vi "GetData.vi"(0 "reference":refnum<class "VdRs232.lvclass">, 1 "stringIn":string, 2 "numberOfBytes(-1=all)":i32=-1, 3 "timeOut(-1ms=ignored)":i32=-1, 4 "MatchPatternToIndicateCompleteResponse(Use default if not wired)":string, 5 "error in (no error)":errorcluster, 6 "WaitForOtherProcessesToBeFinished(False)":bool, 9 "WaitTimeIfPatternNotFound(20ms)":u32=20) -> (14 "duplicate reference":refnum<class "VdRs232.lvclass">, 15 "wholeString":string, 16 "stringRead":string, 17 "TimedOut":bool, 19 "error out":errorcluster)   [LabVIEW 2020, in "VdRs232.lvclass"]
doc: "Reads data from the com-port"
uses:
  VdRs232.lvclass
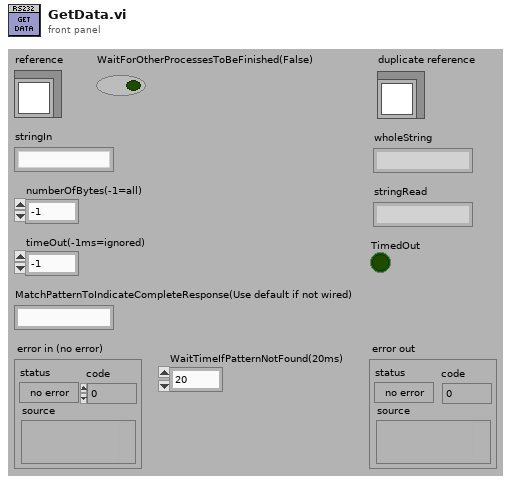
[diagram p1: front panel]
types:
  T1 = typedef "VdRs232.lvclass/ObjectAttributes.ctl" = cluster{"visaRef":refnum<visa-resource-name>, "portSetting":T2, "TimeoutTime(ms)":u32, "TerminationCharUsed":bool, "MatchPatternToIndicateCompleteResponse":string, "Creators":i32, "EndCharToSendForEveryMessage":string, "DefaultReadDataSize":u32, "SynchronousMode":bool, "Lock":T7}
  T2 = typedef "VdRs232.lvclass/ComParamsType.ctl" = cluster{"portNbr":T3, "baudRate":T4, "flowControl":T5, "parity":T6, "dataBits":u16, "stop bits (10: 1 bit)":u16}
  T3 = typedef "VdRs232.lvclass/VdRs232I_ComPortType.ctl" = enum16{"Com1", "Com2", "Com3", "Com4", "Com5", "Com6", "Com7", "Com8", "Com9", "Com10", "Com11", "Com12", "Com13", "Com14", "Com15", "Com16", "Com17", "Com18", "Com19", "Com20", "Com21", "Com22", "Com23", "Com24", "Com25", "Com26", "Com27", "Com28", "Com29", "Com30", "Com31", "Com32", "Com33", "Com34", "Com35", "Com36", "Com37", "Com38", "Com39", "Com40", "Com41", "Com42", "Com43", "Com44", "Com45", "Com46", "Com47", "Com48", "Com49", "Com50", "Com51", "Com52", "Com53", "Com54", "Com55", "Com56", "Com57", "Com58", "Com59", "Com60", "Com61", "Com62", "Com63", "Com64", "Com65", "Com66", "Com67", "Com68", "Com69", "Com70", "Com71", "Com72", "Com73", "Com74", "Com75", "Com76", "Com77", "Com78", "Com79", "Com80", "Com81", "Com82", "Com83", "Com84", "Com85", "Com86", "Com87", "Com88", "Com89", "Com90", "Com91", "Com92", "Com93", "Com94", "Com95", "Com96", "Com97", "Com98", "Com99", "Com100", "Com101", "Com102", "Com103", "Com104", "Com105", "Com106", "Com107", "Com108", "Com109", "Com110", "Com111", "Com112", "Com113", "Com114", "Com115", "Com116", "Com117", "Com118", "Com119", "Com120", "Com121", "Com122", "Com123", "Com124", "Com125", "Com126", "Com127", "Com128", "Com129", "Com130", "Com131", "Com132", "Com133", "Com134", "Com135", "Com136", "Com137", "Com138", "Com139", "Com140", "Com141", "Com142", "Com143", "Com144", "Com145", "Com146", "Com147", "Com148", "Com149", "Com150", "Com151", "Com152", "Com153", "Com154", "Com155", "Com156", "Com157", "Com158", "Com159", "Com160", "Com161", "Com162", "Com163", "Com164", "Com165", "Com166", "Com167", "Com168", "Com169", "Com170", "Com171", "Com172", "Com173", "Com174", "Com175", "Com176", "Com177", "Com178", "Com179", "Com180", "Com181", "Com182", "Com183", "Com184", "Com185", "Com186", "Com187", "Com188", "Com189", "Com190", "Com191", "Com192", "Com193", "Com194", "Com195", "Com196", "Com197", "Com198", "Com199", "Com200", "Com201", "Com202", "Com203", "Com204", "Com205", "Com206", "Com207", "Com208", "Com209", "Com210", "Com211", "Com212", "Com213", "Com214", "Com215", "Com216", "Com217", "Com218", "Com219", "Com220", "Com221", "Com222", "Com223", "Com224", "Com225", "Com226", "Com227", "Com228", "Com229", "Com230", "Com231", "Com232", "Com233", "Com234", "Com235", "Com236", "Com237", "Com238", "Com239", "Com240", "Com241", "Com242", "Com243", "Com244", "Com245", "Com246", "Com247", "Com248", "Com249", "Com250", "Com251", "Com252", "Com253", "Com254", "Com255"}
  T4 = typedef "VdRs232.lvclass/VdBaudRateType.ctl" = enum16{"1200", "2400", "9600", "14400", "19200", "28800", "38400", "57600", "115200", "230400", "460800", "691200", "921600"}
  T5 = typedef "VdRs232.lvclass/VdFlowControlType.ctl" = enum16{"None", "CTS/RTS", "XOn/XOff"}
  T6 = typedef "VdRs232.lvclass/VdParityType.ctl" = enum16{"None", "Odd", "Even"}
  T7 = typedef "Semaphore RefNum" = refnum<k1>
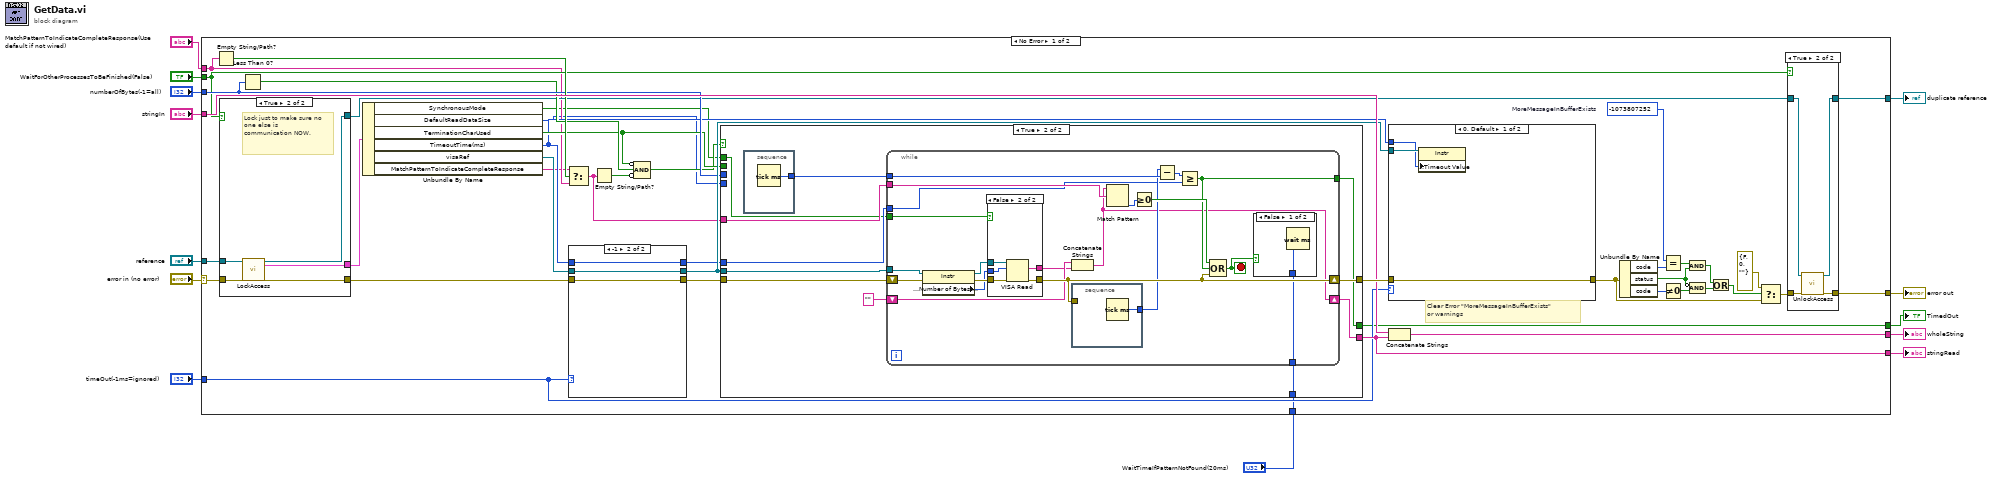
[diagram p0: block diagram]
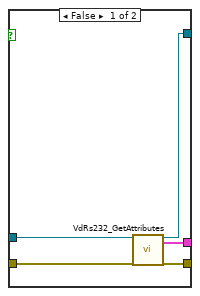
[diagram p3: hidden frame]
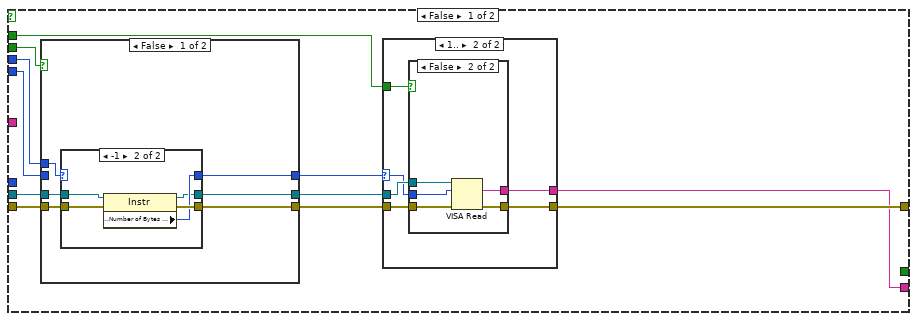
[diagram p4: hidden frame]
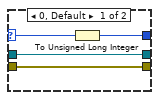
[diagram p5: hidden frame]
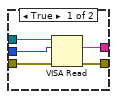
[diagram p8: hidden frame]
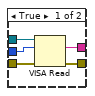
[diagram p9: hidden frame]
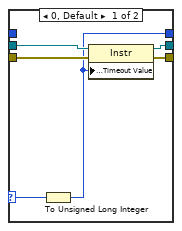
[diagram p12: hidden frame]
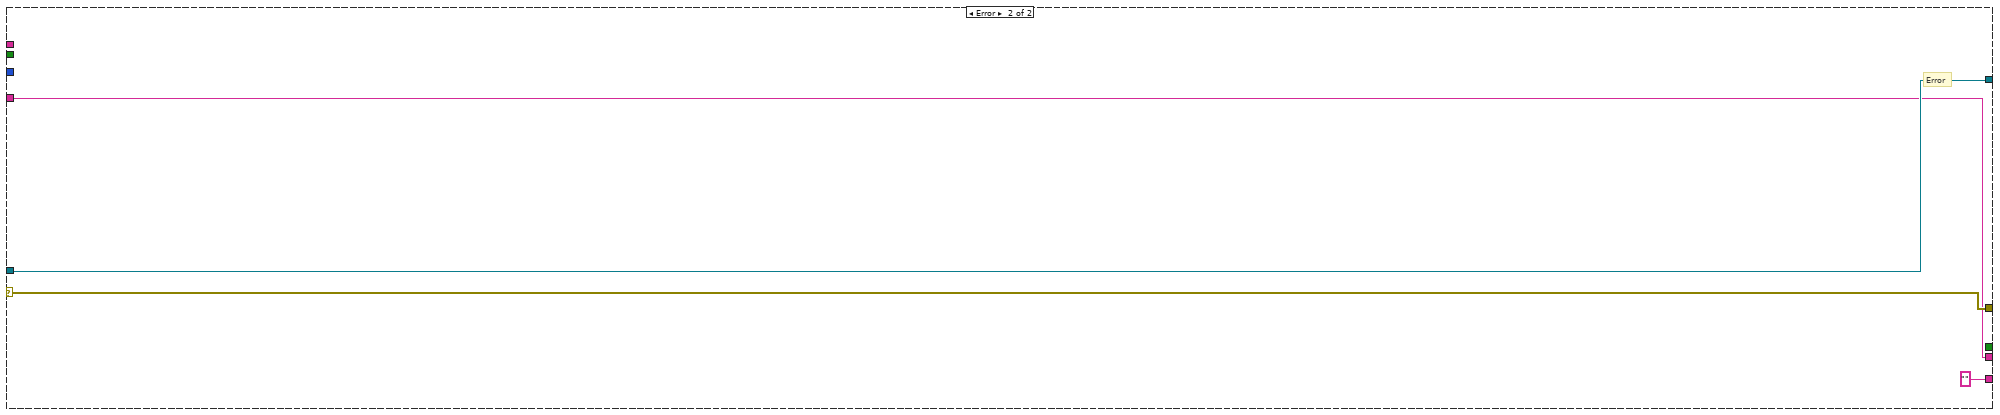
[diagram p13: hidden frame]
diagram:
  n1 = case shown="No Error" "error in (no error)" {
    selector: "error in (no error)" -> [w52 w179]
    tunnel: [w49 w179] -> w13
    tunnel: "reference" -> [w23 w178]
    tunnel: [w21 w178] -> w10
    tunnel: "numberOfBytes(-1=all)" -> [w32 _]
    tunnel: [w46 "" ("read buffer")] -> w7
    tunnel: "timeOut(-1ms=ignored)" -> [w43 _]
    tunnel: "stringIn" -> [w47 w176]
    tunnel: [w45 w176] -> w5
    tunnel: "MatchPatternToIndicateCompleteResponse(Use default if not wired)" -> [w18 _]
    tunnel: [w24 _] -> w3
    tunnel: "WaitForOtherProcessesToBeFinished(False)" -> [w19 _]
    tunnel: "WaitTimeIfPatternNotFound(20ms)" -> [w14 _]
    frame No Error {
      w41 = -1073807252  # MoreMessageInBufferExists
      # "Clear Error \"MoreMessageInBufferExists\"\nor warnings"
      n2 = Empty String/Path?(string/path=w18) -> (empty?=w33:bool)
      n3 = case shown="True" w19 {
        tunnel: w23 -> [w65 w70]
        tunnel: w52 -> [w67 w72]
        tunnel: [w66 w71] -> w51
        tunnel: [w64 w69] -> w22
        tunnel: [w63 w68] -> w20
        frame False {
          n4 = call "VdRs232_GetAttributes.vi"("reference in"=w65, "error in (no error)"=w67) -> ("reference out"=w64:refnum<class "VdRs232.lvclass">, "Data"=w63:T1, "error out"=w66:errorcluster)  [unwired: 1 in, 14 out]
        }
        frame True {
          # "Lock just to make sure no one else is communication NOW."
          n5 = call "LockAccess.vi"("reference in"=w70, "error in (no error)"=w72) -> ("reference out"=w69:refnum<class "VdRs232.lvclass">, "Data"=w68:T1, "error out"=w71:errorcluster)  [unwired: 14 in, 1 out]
        }
      }
      n6 = Less Than 0?(x=w32) -> (x < 0?=w31:bool)
      n7 = Unbundle By Name(w20) -> ("SynchronousMode"=w15:bool, "DefaultReadDataSize"=w16:u32, "TerminationCharUsed"=w30:bool, "TimeoutTime(ms)"=w26:u32, "visaRef"=w48:refnum<visa-resource-name>, "MatchPatternToIndicateCompleteResponse"=w17:string)
      n8 = Select(t=w17, s=w33, f=w18) -> (s? t:f=w28:string)
      n9 = case shown="-1" w43 {
        selector: w43 -> [w168 _]
        tunnel: [w172 w175] -> w56
        tunnel: w51 -> [w171 w175]
        tunnel: [w170 w174] -> w44
        tunnel: w48 -> [w169 w174]
        tunnel: w26 -> [_ w173]
        tunnel: [w167 w173] -> w25
        frame 0, Default {
          n10 = To Unsigned Long Integer(number=w168) -> (unsigned 32bit integer=w167:u32)
          n11 = property class="Instr"(reference=w169, error in=w171, "General Settings:Timeout Value"=w167) -> (reference out=w170:refnum<visa-resource-name>, error out=w172:errorcluster)
        }
        frame -1 {
        }
      }
      n12 = Empty String/Path?(string/path=w28) -> (empty?=w27:bool)
      n13 = Compound Arithmetic op=AND(invert w30, w31, invert w27) -> (w29:bool)
      n14 = case shown="True" w29 {
        tunnel: w56 -> [w83 w128]
        tunnel: [w80 w125] -> w46
        tunnel: [w81 w129] -> w55
        tunnel: w44 -> [w77 w124]
        tunnel: w32 -> [w76 _]
        tunnel: w30 -> [w75 _]
        tunnel: w28 -> [_ w123]
        tunnel: w25 -> [_ w122]
        tunnel: [_ w121] -> w24
        tunnel: w16 -> [w74 _]
        tunnel: w15 -> [w73 w120]
        tunnel: w14 -> [_ w119]
        frame False {
          n15 = case shown="False" w75 {
            tunnel: w83 -> [w89 w101]
            tunnel: w76 -> [w87 _]
            tunnel: [w86 w100] -> w79
            tunnel: [w88 w101] -> w82
            tunnel: [w85 w99] -> w78
            tunnel: w77 -> [w84 w100]
            tunnel: w74 -> [_ w99]
            frame False {
              n16 = case shown="-1" w87 {
                selector: w87 -> [w91 _]
                tunnel: w84 -> [w92 w96]
                tunnel: w89 -> [w93 w98]
                tunnel: [w90 w95] -> w85
                tunnel: [w92 w94] -> w86
                tunnel: [w93 w97] -> w88
                frame 0, Default {
                  n17 = To Unsigned Long Integer(number=w91) -> (unsigned 32bit integer=w90:u32)
                }
                frame -1 {
                  n18 = property class="Instr"(reference=w96, error in=w98) -> (reference out=w94:refnum<visa-resource-name>, error out=w97:errorcluster, "Serial Settings:Number of Bytes at Serial Port"=w95:u32)
                }
              }
            }
            frame True {
              # "Since we're looking for\nTermChar anyway, we might\nas well set this to highest\npossible number. We either\nfind the character, or we\ncrash. Setting the buffer\nto a large size could help too."
            }
          }
          n19 = case shown="1.." w78 {
            selector: w78 -> [_ w104]
            tunnel: w79 -> [_ w106]
            tunnel: w82 -> [w102 w108]
            tunnel: [w102 w107] -> w81
            tunnel: [_ w105] -> w80
            tunnel: w73 -> [_ w103]
            frame 0, Default {
            }
            frame 1.. {
              n20 = case shown="False" w103 {
                tunnel: w106 -> [w111 w116]
                tunnel: w108 -> [w113 w118]
                tunnel: [w112 w117] -> w107
                tunnel: [w110 w115] -> w105
                tunnel: w104 -> [w109 w114]
                frame True {
                  n21 = VISA Read(VISA resource name=w111, byte count=w109, error in (no error)=w113) -> (read buffer=w110:string, error out=w112:errorcluster)  [unwired: 2 out]
                }
                frame False {
                  n22 = VISA Read(VISA resource name=w116, byte count=w114, error in (no error)=w118) -> (read buffer=w115:string, error out=w117:errorcluster)  [unwired: 2 out]
                }
              }
            }
          }
        }
        frame True {
          n23 = stacked-sequence {
            tunnel: [w130] -> w126
            frame #0 {
              n24 = Tick Count (ms)() -> (millisecond timer value=w130:u32)
            }
          }
          n25 = while {
            shift-right: [w134] -> w125
            shift-left: "" ("wholeString") -> [w136]
            shift-right: [w148] -> w129
            shift-left: w128 -> [w150]
            tunnel: w124 -> [w139]
            tunnel: w123 -> [w145]
            tunnel: w126 -> [w147]
            tunnel: [w142] -> w121
            tunnel: w122 -> [w133]
            tunnel: w120 -> [w132]
            tunnel: w119 -> [w131]
            stop <- w141 stop-if-true
            n26 = property class="Instr"(reference=w139, error in=w150) -> (reference out=w138:refnum<visa-resource-name>, error out=w149:errorcluster, "Serial Settings:Number of Bytes at Serial Port"=w137:u32)
            n27 = case shown="False" w132 {
              tunnel: [w155 w160] -> w148
              tunnel: w138 -> [w153 w158]
              tunnel: w137 -> [w152 w157]
              tunnel: [w151 w156] -> w135
              tunnel: w149 -> [w154 w159]
              frame True {
                n28 = VISA Read(VISA resource name=w153, byte count=w152, error in (no error)=w154) -> (read buffer=w151:string, error out=w155:errorcluster)  [unwired: 2 out]
              }
              frame False {
                n29 = VISA Read(VISA resource name=w158, byte count=w157, error in (no error)=w159) -> (read buffer=w156:string, error out=w160:errorcluster)  [unwired: 2 out]
              }
            }
            n30 = Concatenate Strings(w136, w135) -> (w134:string)
            n31 = stacked-sequence {
              tunnel: [w161] -> w140
              tunnel: w148 -> [_]
              frame #0 {
                n32 = Tick Count (ms)() -> (millisecond timer value=w161:u32)
              }
            }
            n33 = Match Pattern(string=w134, regular expression=w145) -> (offset past match=w144:i32)  [unwired: 4 out]
            n34 = Greater Or Equal To 0?(x=w144) -> (x >= 0?=w143:bool)
            n35 = Subtract(x=w140, y=w147) -> (x-y=w146:u32)
            n36 = Greater Or Equal?(x=w146, y=w133) -> (x >= y?=w142:bool)
            n37 = Compound Arithmetic op=OR(w143, w142, w148) -> (w141:bool)
            n38 = case shown="False" w141 {
              tunnel: w131 -> [w162 _]
              frame False {
                n39 = Wait (ms)(milliseconds to wait=w162) -> ()  [unwired: 1 out]
              }
              frame True {
              }
            }
          }
        }
      }
      n40 = case shown="0, Default" w43 {
        tunnel: [w165 w166] -> w54
        tunnel: w55 -> [w165 w166]
        tunnel: w44 -> [w164 _]
        tunnel: w26 -> [w163 _]
        frame 0, Default {
          n41 = property class="Instr"(reference=w164, "General Settings:Timeout Value"=w163) -> ()  [unwired: 1 in, 2 out]
        }
        frame -1 {
        }
      }
      n42 = Concatenate Strings(w47, w46) -> (w45:string)
      n43 = Unbundle By Name(w54) -> ("code"=w42:i32, "status"=w39:bool, "code"=w37:i32)
      n44 = Equal?(x=w41, y=w42) -> (x = y?=w40:bool)
      n45 = Not Equal To 0?(x=w37) -> (x != 0?=w36:bool)
      n46 = And(x=w40, y=w39) -> (x .and. y?=w34:bool)
      n47 = Compound Arithmetic op=AND(invert w39, w36) -> (w35:bool)
      n48 = Or(x=w34, y=w35) -> (x .or. y?=w38:bool)
      n49 = Select(t=errorcluster {"status"=FALSE, "code"=0, "source"=""}, s=w38, f=w54) -> (s? t:f=w50:errorcluster)
      n50 = case shown="True" w19 {
        tunnel: w22 -> [w57 w60]
        tunnel: w50 -> [w58 w62]
        tunnel: [w58 w61] -> w49
        tunnel: [w57 w59] -> w21
        frame False {
        }
        frame True {
          n51 = call "UnlockAccess.vi"("reference in"=w60, "error in (no error)"=w62) -> ("reference out"=w59:refnum<class "VdRs232.lvclass">, "error out"=w61:errorcluster)  [unwired: 16 in]
        }
      }
    }
    frame Error {
      # "Error"
    }
  }
  "error out" <- w13
  "duplicate reference" <- w10
  "wholeString" <- w5
  "stringRead" <- w7
  "TimedOut" <- w3
